vi "Car Wash.vi"() -> ()   [LabVIEW 2017]
uses:
  Bundyra/support/Message Queue/Message Queue.lvlib
  Bundyra/Boiler/Boiler.lvlib
  <vilib>/Utility/error.llb/Error Cluster From Error Code.vi
  <vilib>/ErrorRing/Error Ring.xnode
  Bundyra/Boiler/Boiler References.ctl
  Car Wash Data.ctl
  Bundyra/support/Message Queue/Message Cluster.ctl
  Bundyra/support/Message Queue/All Message Queues.ctl
  Bundyra/Boiler/Boiler Configuration.ctl
  Notifiers.ctl
panel:
  in  "Notifiers":T1
  in  "Boiler Configuration":T2
  in  "Message Queues":T3
  in  "error in":errorcluster
  out "error out":errorcluster
  in  "Simulate Failure":bool
  out "Vehicle Postion":bool
  out "Air Dry":bool
  out "Tire Shine Foam":bool
  out "Spot Free Rinse":bool
  out "Low Pressure  Wax":bool
  out "High Pressure Wash":bool
  out "Pre-soak":bool
  out "Bug Remover":bool
  out "Under Body Wash":bool
  # "Wash entry"
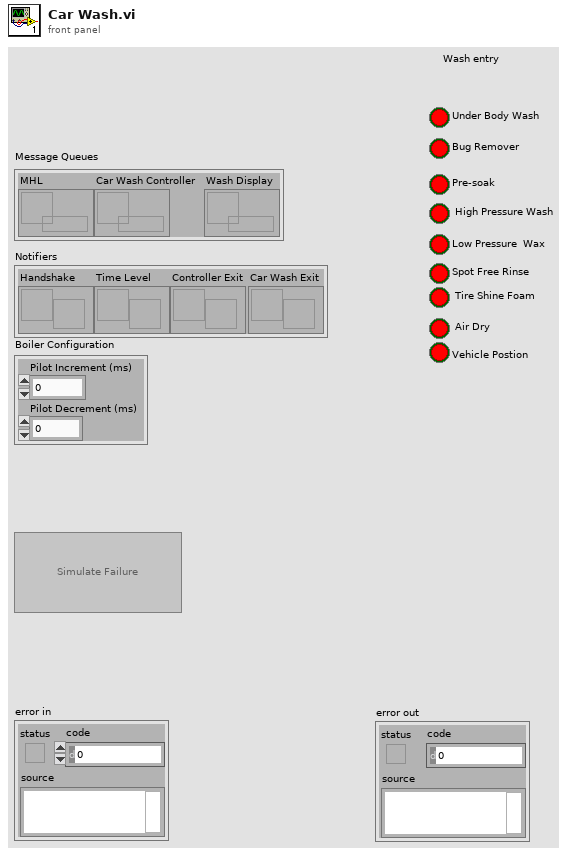
[diagram p1: front panel]
types:
  T1 = typedef "Notifiers.ctl" = cluster{"Handshake":refnum<notifier>, "Time Level":refnum<notifier>, "Controller Exit":refnum<notifier>, "Car Wash Exit":refnum<notifier>}
  T2 = typedef "Boiler.lvlib/Boiler Configuration.ctl" = cluster{"Pilot Increment (ms)":u32, "Pilot Decrement (ms)":u32}
  T3 = typedef "Message Queue.lvlib/All Message Queues.ctl" = cluster{"MHL":refnum<queue>, "Car Wash Controller":refnum<queue>, "Wash Display":refnum<queue>}
  T4 = typedef "Boiler.lvlib/Car Wash Data.ctl" = cluster{"Car Wash  References":T5, "Under Body Wash":bool, "Bug Remover":bool, "Pre-soak":bool, " High Pressure Wash":bool, "Low Pressure  Wax":bool, "Spot Free Rinse":bool, " Tire Shine Foam":bool, " Air Dry":bool, "Vehicle Position":bool}
  T5 = typedef "Boiler.lvlib/Boiler References.ctl" = cluster{"Simulate Failure":refnum<vi>}
  T6 = enum8{"Enabled", "Disabled", "Disabled and Grayed Out"}
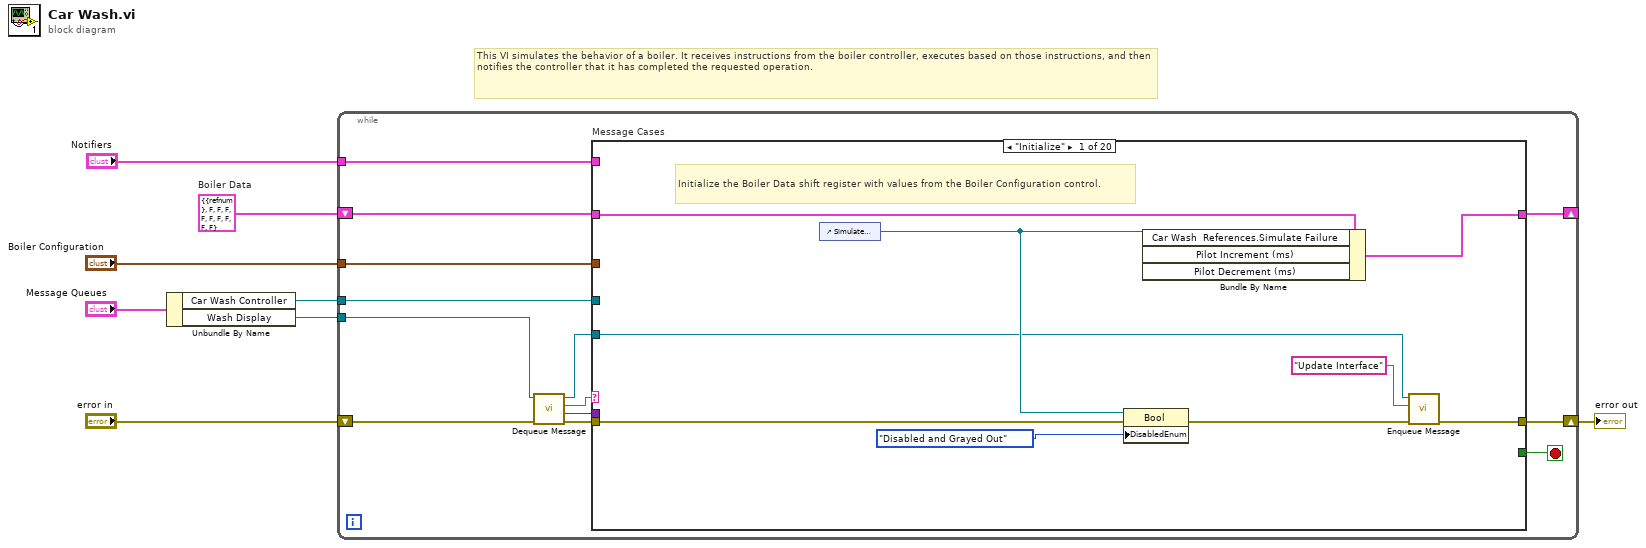
[diagram p0: block diagram]
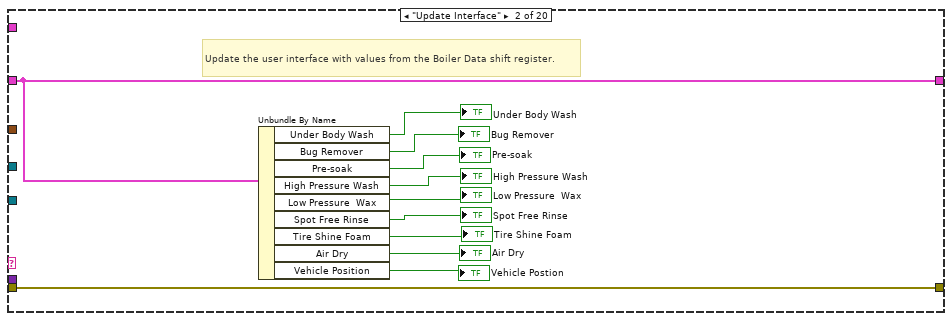
[diagram p2: hidden frame]
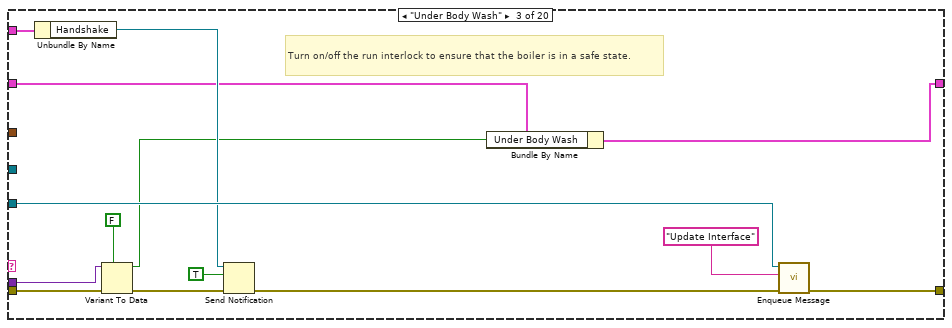
[diagram p3: hidden frame]
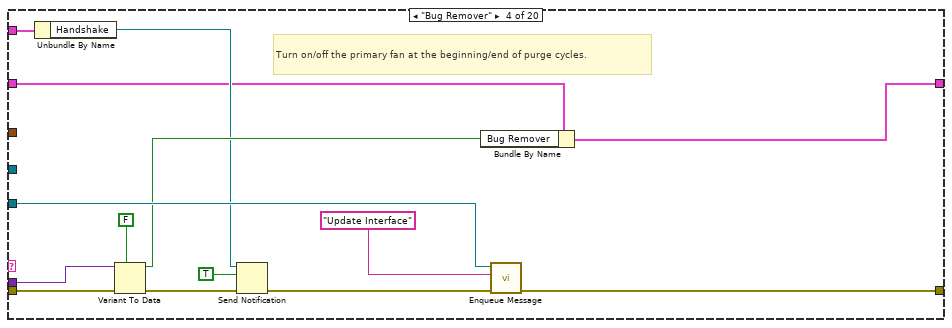
[diagram p4: hidden frame]
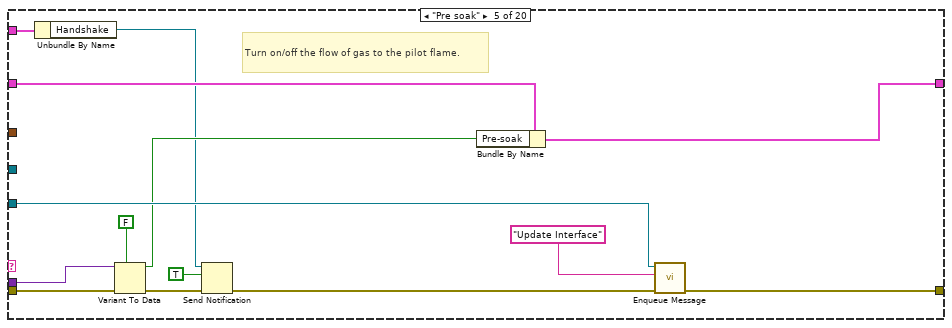
[diagram p5: hidden frame]
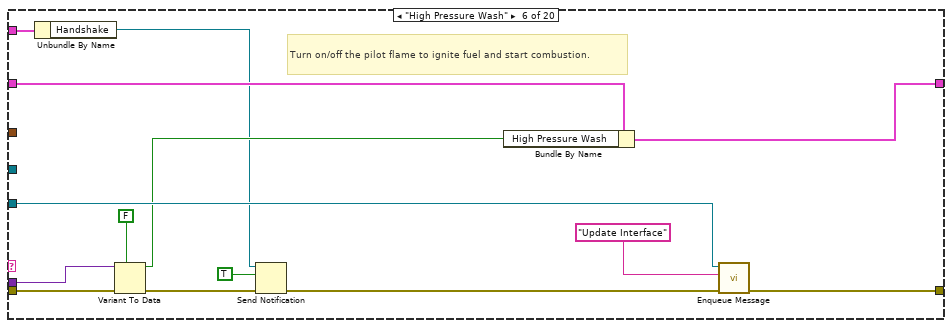
[diagram p6: hidden frame]
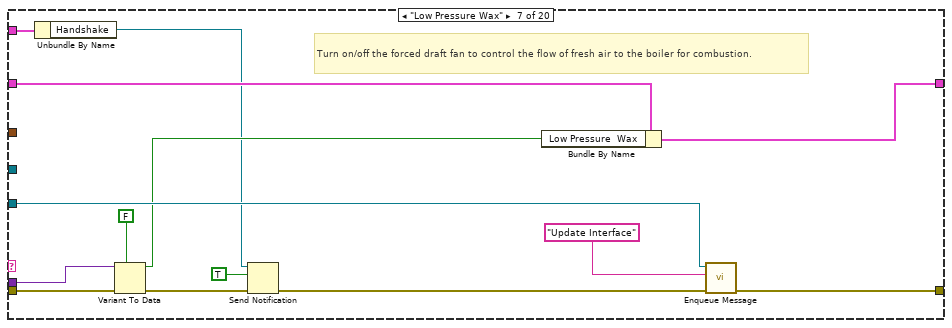
[diagram p7: hidden frame]
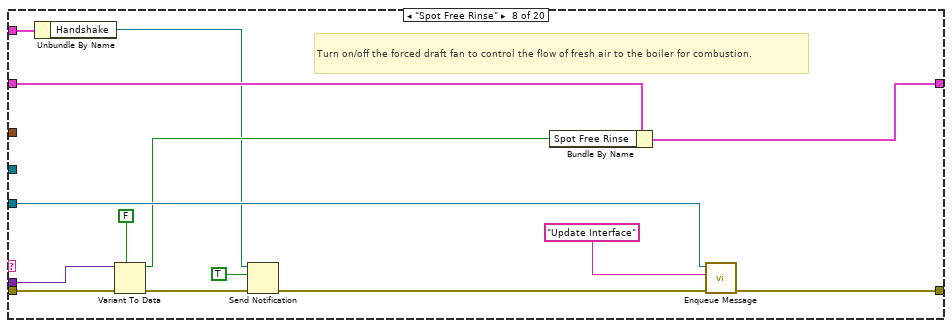
[diagram p8: hidden frame]
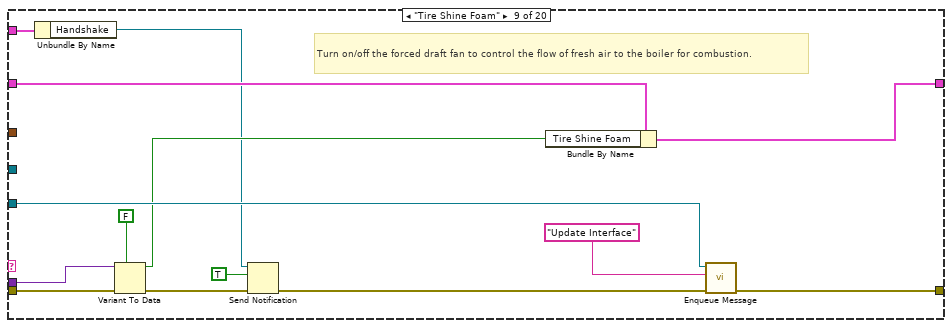
[diagram p9: hidden frame]
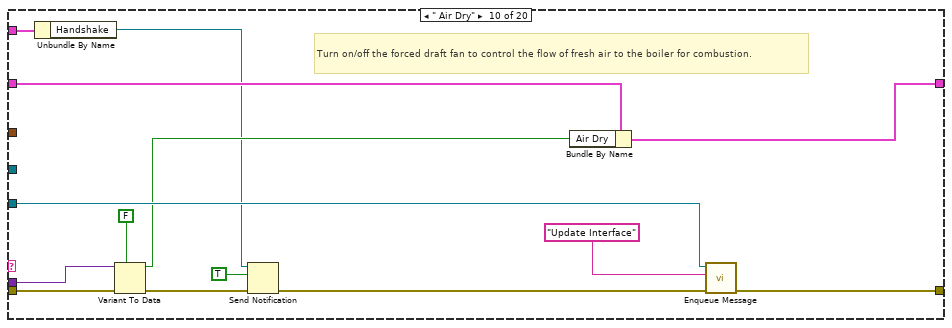
[diagram p10: hidden frame]
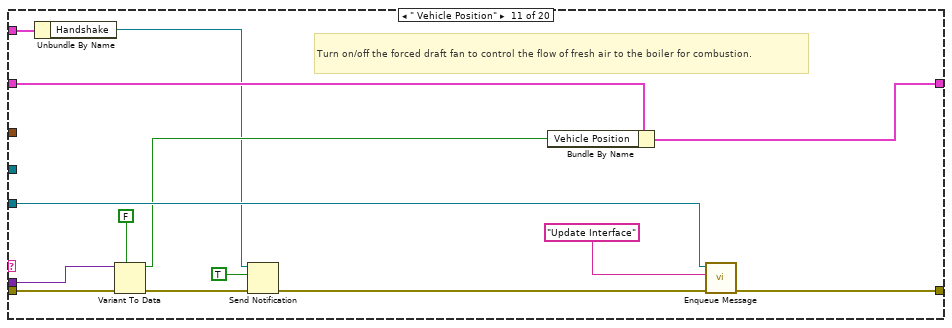
[diagram p11: hidden frame]
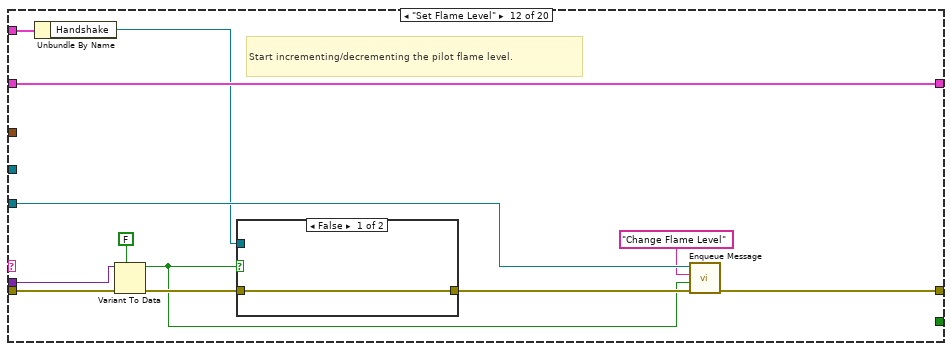
[diagram p12: hidden frame]
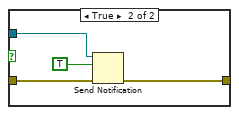
[diagram p13: hidden frame]
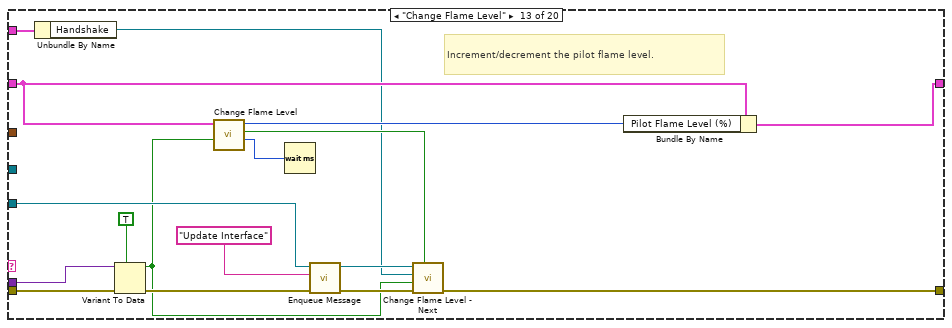
[diagram p14: hidden frame]
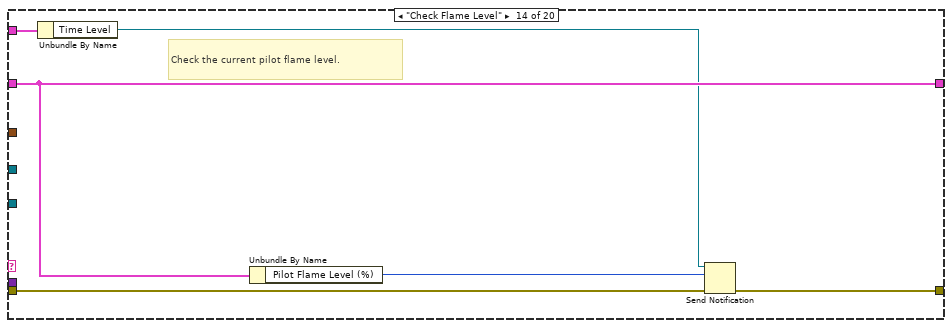
[diagram p15: hidden frame]
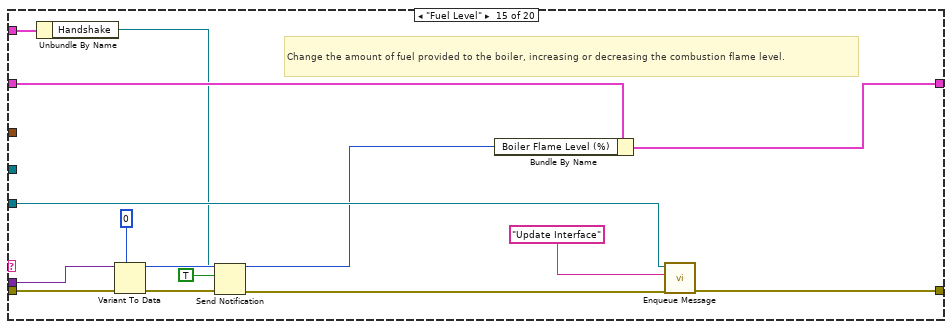
[diagram p16: hidden frame]
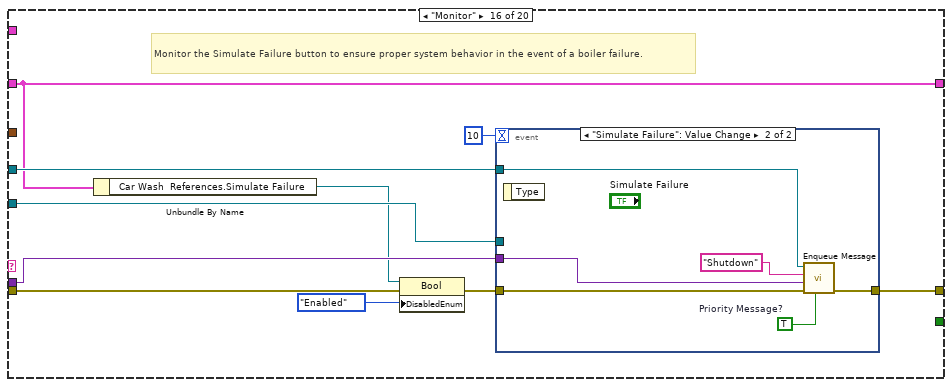
[diagram p17: hidden frame]
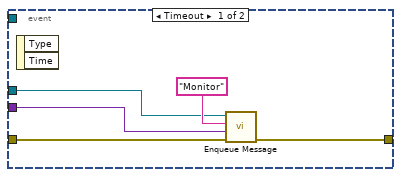
[diagram p18: hidden frame]
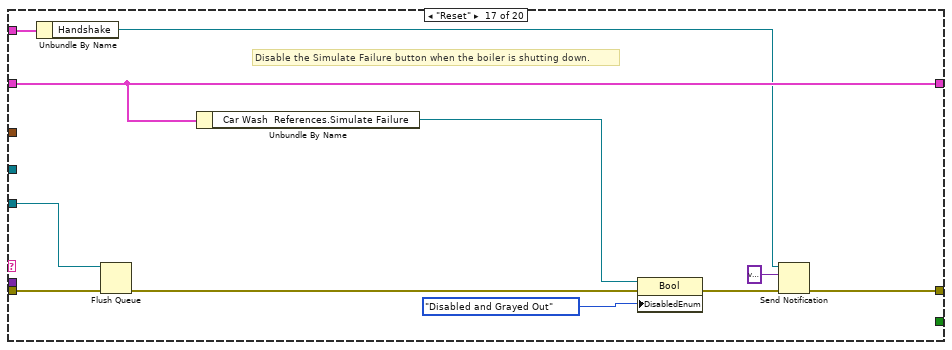
[diagram p19: hidden frame]
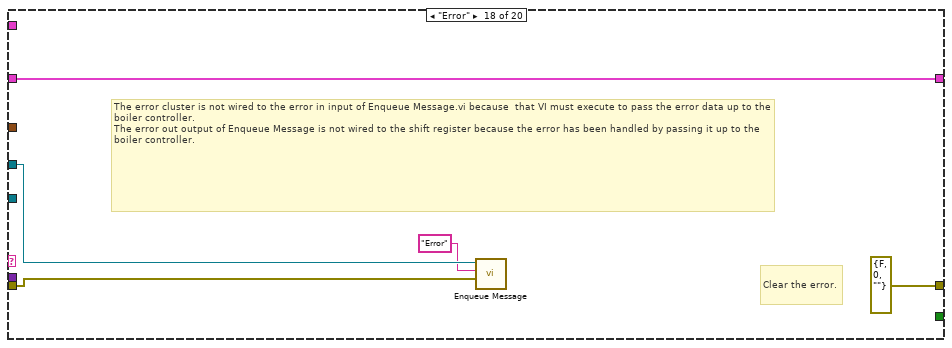
[diagram p20: hidden frame]
diagram:
  w7 = T4 {"Car Wash  References"={"Simulate Failure"=refnum}, "Under Body Wash"=FALSE, "Bug Remover"=FALSE, "Pre-soak"=FALSE, " High Pressure Wash"=FALSE, "Low Pressure  Wax"=FALSE, "Spot Free Rinse"=FALSE, " Tire Shine Foam"=FALSE, " Air Dry"=FALSE, "Vehicle Position"=FALSE}  # Boiler Data
  # "This VI simulates the behavior of a boiler. It receives instructions from the boiler controller, executes based on those instructions, and then notifies the controller that it has completed the requested operation."
  n1 = Unbundle By Name("Message Queues") -> ("Car Wash Controller"=w4:refnum<queue>, "Wash Display"=w3:refnum<queue>)
  n2 = while {
    tunnel: w3 -> [w12]
    shift-right: [w20] -> _
    shift-left: w7 -> [w21]
    shift-right: [w18] -> w8
    shift-left: "error in" -> [w17]
    tunnel: w4 -> [w11]
    tunnel: "Notifiers" -> [w10]
    tunnel: "Boiler Configuration" -> [w9]
    stop <- w19 stop-if-true
    n3 = call "Dequeue Message.vi"("error in (no error)"=w17, "Message Queue"=w12) -> ("error out"=w16:errorcluster, "Message Data"=w14:variant, "Message"=w15:string, "dup Message Queue"=w13:refnum<queue>)  [unwired: 6 in]
    n4 = case "Message Cases" shown="\"Initialize\"" w15 {
      selector: w15 -> [_ _ _ _ _ _ _ _ _ _ _ _ _ _ _ _ _ _ _ w269]
      tunnel: w13 -> [w24 _ w55 w65 w79 w93 w107 w121 w135 w149 w163 w177 w198 _ w218 w230 w250 _ w267 _]
      tunnel: w16 -> [w23 w41 w54 w67 w81 w95 w109 w123 w137 w151 w165 w174 w200 w204 w220 w222 w249 w255 w264 w275]
      tunnel: [w25 w41 w49 w61 w73 w87 w101 w115 w129 w143 w157 w178 w189 w207 w211 w223 w247 errorcluster {"status"=FALSE, "code"=0, "source"=""} ("error out") w263 w274] -> w18
      tunnel: w21 -> [w28 w40 w44 w57 w78 w92 w106 w120 w134 w148 w162 w179 w197 w206 w216 w224 w252 w258 w266 w276]
      tunnel: [w29 w40 w42 w56 w77 w91 w104 w118 w132 w146 w160 w179 w196 w206 w214 w224 w252 w258 w266 w276] -> w20
      tunnel: [_ _ _ _ _ _ _ _ _ _ _ _ _ _ _ _ _ _ TRUE _] -> w19
      tunnel: w14 -> [_ _ w52 w66 w80 w94 w108 w122 w136 w150 w164 w173 w199 _ w219 w228 _ _ _ _]
      tunnel: w11 -> [_ _ _ _ _ _ _ _ _ _ _ _ _ _ _ w229 _ w257 _ _]
      tunnel: w10 -> [_ _ w47 w60 w72 w86 w100 w114 w128 w142 w156 w169 w188 w205 w210 _ w246 _ w262 w272]
      tunnel: w9 -> [_ _ _ _ _ _ _ _ _ _ _ _ _ _ _ _ _ _ _ _]
      frame "Initialize" {
        # "Initialize the Boiler Data shift register with values from the Boiler Configuration control."
        n5 = control-ref of="Simulate Failure"() -> (w27:refnum<vi>)
        n6 = property class="Bool"(reference=w27, error in=w23, "DisabledEnum"=T6."Disabled and Grayed Out" ("Disabled")) -> (error out=w22:errorcluster)  [unwired: 1 out]
        n7 = Bundle By Name(cluster=w28, "Car Wash  References.Simulate Failure"=w27) -> (w29:T4)  [unwired: 2 in]
        n8 = call "Enqueue Message.vi"("error in (no error)"=w22, "Message"="Update Interface", "Message Queue"=w24) -> ("error out"=w25:errorcluster)  [unwired: 7 in, 1 out]
      }
      frame "Update Interface" {
        # "Update the user interface with values from the Boiler Data shift register."
        n9 = Unbundle By Name(w40) -> ("Under Body Wash"=→"Under Body Wash":bool, "Bug Remover"=→"Bug Remover":bool, "Pre-soak"=→"Pre-soak":bool, "High Pressure Wash"=→"High Pressure Wash":bool, "Low Pressure  Wax"=→"Low Pressure  Wax":bool, "Spot Free Rinse"=→"Spot Free Rinse":bool, "Tire Shine Foam"=→"Tire Shine Foam":bool, "Air Dry"=→"Air Dry":bool, "Vehicle Position"=→"Vehicle Postion":bool)
      }
      frame "Under Body Wash" {
        # "Turn on/off the run interlock to ensure that the boiler is in a safe state."
        n10 = Unbundle By Name(w47) -> ("Handshake"=w45:refnum<notifier>)
        n11 = Variant To Data(error in=w54, type=FALSE ("Run Interlock"), Variant=w52) -> (data=w43:bool, error out=w50:errorcluster)
        n12 = Send Notification(notification=TRUE, notifier=w45, error in (no error)=w50) -> (error out=w48:errorcluster)  [unwired: 1 out]
        n13 = Bundle By Name(cluster=w44, "Under Body Wash"=w43) -> (w42:T4)
        n14 = call "Enqueue Message.vi"("error in (no error)"=w48, "Message"="Update Interface", "Message Queue"=w55) -> ("error out"=w49:errorcluster)  [unwired: 7 in, 1 out]
      }
      frame "Bug Remover" {
        # "Turn on/off the primary fan at the beginning/end of purge cycles."
        n15 = Unbundle By Name(w60) -> ("Handshake"=w58:refnum<notifier>)
        n16 = Variant To Data(error in=w67, type=FALSE ("Run Interlock"), Variant=w66) -> (data=w64:bool, error out=w63:errorcluster)
        n17 = Send Notification(notification=TRUE ("Run Interlock"), notifier=w58, error in (no error)=w63) -> (error out=w62:errorcluster)  [unwired: 1 out]
        n18 = Bundle By Name(cluster=w57, "Bug Remover"=w64) -> (w56:T4)
        n19 = call "Enqueue Message.vi"("error in (no error)"=w62, "Message"="Update Interface", "Message Queue"=w65) -> ("error out"=w61:errorcluster)  [unwired: 7 in, 1 out]
      }
      frame "Pre soak" {
        # "Turn on/off the flow of gas to the pilot flame."
        n20 = Unbundle By Name(w72) -> ("Handshake"=w70:refnum<notifier>)
        n21 = Variant To Data(error in=w81, type=FALSE ("Run Interlock"), Variant=w80) -> (data=w76:bool, error out=w75:errorcluster)
        n22 = Send Notification(notification=TRUE ("Run Interlock"), notifier=w70, error in (no error)=w75) -> (error out=w74:errorcluster)  [unwired: 1 out]
        n23 = Bundle By Name(cluster=w78, "Pre-soak"=w76) -> (w77:T4)
        n24 = call "Enqueue Message.vi"("error in (no error)"=w74, "Message"="Update Interface", "Message Queue"=w79) -> ("error out"=w73:errorcluster)  [unwired: 7 in, 1 out]
      }
      frame "High Pressure Wash" {
        # "Turn on/off the pilot flame to ignite fuel and start combustion."
        n25 = Unbundle By Name(w86) -> ("Handshake"=w84:refnum<notifier>)
        n26 = Variant To Data(error in=w95, type=FALSE ("Run Interlock"), Variant=w94) -> (data=w90:bool, error out=w89:errorcluster)
        n27 = Send Notification(notification=TRUE ("Run Interlock"), notifier=w84, error in (no error)=w89) -> (error out=w88:errorcluster)  [unwired: 1 out]
        n28 = Bundle By Name(cluster=w92, "High Pressure Wash"=w90) -> (w91:T4)
        n29 = call "Enqueue Message.vi"("error in (no error)"=w88, "Message"="Update Interface", "Message Queue"=w93) -> ("error out"=w87:errorcluster)  [unwired: 7 in, 1 out]
      }
      frame "Low Pressure Wax" {
        # "Turn on/off the forced draft fan to control the flow of fresh air to the boiler for combustion."
        n30 = Unbundle By Name(w100) -> ("Handshake"=w98:refnum<notifier>)
        n31 = Variant To Data(error in=w109, type=FALSE ("Run Interlock"), Variant=w108) -> (data=w105:bool, error out=w103:errorcluster)
        n32 = Send Notification(notification=TRUE ("Run Interlock"), notifier=w98, error in (no error)=w103) -> (error out=w102:errorcluster)  [unwired: 1 out]
        n33 = Bundle By Name(cluster=w106, "Low Pressure  Wax"=w105) -> (w104:T4)
        n34 = call "Enqueue Message.vi"("error in (no error)"=w102, "Message"="Update Interface", "Message Queue"=w107) -> ("error out"=w101:errorcluster)  [unwired: 7 in, 1 out]
      }
      frame "Spot Free Rinse" {
        # "Turn on/off the forced draft fan to control the flow of fresh air to the boiler for combustion."
        n35 = Unbundle By Name(w114) -> ("Handshake"=w112:refnum<notifier>)
        n36 = Variant To Data(error in=w123, type=FALSE ("Run Interlock"), Variant=w122) -> (data=w119:bool, error out=w117:errorcluster)
        n37 = Send Notification(notification=TRUE ("Run Interlock"), notifier=w112, error in (no error)=w117) -> (error out=w116:errorcluster)  [unwired: 1 out]
        n38 = Bundle By Name(cluster=w120, "Spot Free Rinse"=w119) -> (w118:T4)
        n39 = call "Enqueue Message.vi"("error in (no error)"=w116, "Message"="Update Interface", "Message Queue"=w121) -> ("error out"=w115:errorcluster)  [unwired: 7 in, 1 out]
      }
      frame "Tire Shine Foam" {
        # "Turn on/off the forced draft fan to control the flow of fresh air to the boiler for combustion."
        n40 = Unbundle By Name(w128) -> ("Handshake"=w126:refnum<notifier>)
        n41 = Variant To Data(error in=w137, type=FALSE ("Run Interlock"), Variant=w136) -> (data=w133:bool, error out=w131:errorcluster)
        n42 = Send Notification(notification=TRUE ("Run Interlock"), notifier=w126, error in (no error)=w131) -> (error out=w130:errorcluster)  [unwired: 1 out]
        n43 = Bundle By Name(cluster=w134, "Tire Shine Foam"=w133) -> (w132:T4)
        n44 = call "Enqueue Message.vi"("error in (no error)"=w130, "Message"="Update Interface", "Message Queue"=w135) -> ("error out"=w129:errorcluster)  [unwired: 7 in, 1 out]
      }
      frame " Air Dry" {
        # "Turn on/off the forced draft fan to control the flow of fresh air to the boiler for combustion."
        n45 = Unbundle By Name(w142) -> ("Handshake"=w140:refnum<notifier>)
        n46 = Variant To Data(error in=w151, type=FALSE ("Run Interlock"), Variant=w150) -> (data=w147:bool, error out=w145:errorcluster)
        n47 = Send Notification(notification=TRUE ("Run Interlock"), notifier=w140, error in (no error)=w145) -> (error out=w144:errorcluster)  [unwired: 1 out]
        n48 = Bundle By Name(cluster=w148, "Air Dry"=w147) -> (w146:T4)
        n49 = call "Enqueue Message.vi"("error in (no error)"=w144, "Message"="Update Interface", "Message Queue"=w149) -> ("error out"=w143:errorcluster)  [unwired: 7 in, 1 out]
      }
      frame " Vehicle Position" {
        # "Turn on/off the forced draft fan to control the flow of fresh air to the boiler for combustion."
        n50 = Unbundle By Name(w156) -> ("Handshake"=w154:refnum<notifier>)
        n51 = Variant To Data(error in=w165, type=FALSE ("Run Interlock"), Variant=w164) -> (data=w161:bool, error out=w159:errorcluster)
        n52 = Send Notification(notification=TRUE ("Run Interlock"), notifier=w154, error in (no error)=w159) -> (error out=w158:errorcluster)  [unwired: 1 out]
        n53 = Bundle By Name(cluster=w162, "Vehicle Position"=w161) -> (w160:T4)
        n54 = call "Enqueue Message.vi"("error in (no error)"=w158, "Message"="Update Interface", "Message Queue"=w163) -> ("error out"=w157:errorcluster)  [unwired: 7 in, 1 out]
      }
      frame "Set Flame Level" {
        # "Start incrementing/decrementing the pilot flame level."
        n55 = Unbundle By Name(w169) -> ("Handshake"=w168:refnum<notifier>)
        n56 = Variant To Data(error in=w174, type=FALSE ("Run Interlock"), Variant=w173) -> (data=w170:bool, error out=w172:errorcluster)
        n57 = case shown="False" w170 {
          tunnel: w172 -> [w180 w184]
          tunnel: [w180 w183] -> w171
          tunnel: w168 -> [_ w181]
          frame False {
          }
          frame True {
            n58 = Send Notification(notification=TRUE ("Run Interlock"), notifier=w181, error in (no error)=w184) -> (error out=w183:errorcluster)  [unwired: 1 out]
          }
        }
        n59 = call "Enqueue Message.vi"("error in (no error)"=w171, "Message Data"=w170, "Message"="Change Flame Level", "Message Queue"=w177) -> ("error out"=w178:errorcluster)  [unwired: 6 in, 1 out]
      }
      frame "Change Flame Level" {
        # "Increment/decrement the pilot flame level."
        n60 = Unbundle By Name(w188) -> ("Handshake"=w186:refnum<notifier>)
        n61 = Variant To Data(error in=w200, type=TRUE, Variant=w199) -> (data=w185:bool, error out=w192:errorcluster)
        n62 = call "Change Flame Level.vi"("Increment?"=w185, "Boiler Data"=w197) -> ("Time Increment"=w193:u32, "Limit?"=w187:bool, "Flame Level"=w194:u32)  [unwired: 7 in]
        n63 = Wait (ms)(milliseconds to wait=w193) -> ()  [unwired: 1 out]
        n64 = call "Enqueue Message.vi"("error in (no error)"=w192, "Message"="Update Interface", "Message Queue"=w198) -> ("error out"=w190:errorcluster, "dup Message Queue"=w191:refnum<queue>)  [unwired: 7 in]
        n65 = call "Change Flame Level - Next.vi"("Limit?"=w187, "error in"=w190, "Increment?"=w185, "Handshake"=w186, "Boiler Queue in"=w191) -> ("error out"=w189:errorcluster)  [unwired: 6 in]
        n66 = Bundle By Name(cluster=w197, "Pilot Flame Level (%)"=w194) -> (w196:T4)
      }
      frame "Check Flame Level" {
        # "Check the current pilot flame level."
        n67 = Unbundle By Name(w205) -> ("Time Level"=w202:refnum<notifier>)
        n68 = Unbundle By Name(w206) -> ("Pilot Flame Level (%)"=w203:u32)
        n69 = Send Notification(notification=w203, notifier=w202, error in (no error)=w204) -> (error out=w207:errorcluster)  [unwired: 1 out]
      }
      frame "Fuel Level" {
        # "Change the amount of fuel provided to the boiler, increasing or decreasing the combustion flame level."
        n70 = Unbundle By Name(w210) -> ("Handshake"=w208:refnum<notifier>)
        n71 = Variant To Data(error in=w220, type=u32 0, Variant=w219) -> (data=w215:u32, error out=w213:errorcluster)
        n72 = Send Notification(notification=TRUE ("Run Interlock"), notifier=w208, error in (no error)=w213) -> (error out=w212:errorcluster)  [unwired: 1 out]
        n73 = Bundle By Name(cluster=w216, "Boiler Flame Level (%)"=w215) -> (w214:T4)
        n74 = call "Enqueue Message.vi"("error in (no error)"=w212, "Message"="Update Interface", "Message Queue"=w218) -> ("error out"=w211:errorcluster)  [unwired: 7 in, 1 out]
      }
      frame "Monitor" {
        # "Monitor the Simulate Failure button to ensure proper system behavior in the event of a boiler failure."
        n75 = Unbundle By Name(w224) -> ("Car Wash  References.Simulate Failure"=w227:refnum<vi>)
        n76 = property class="Bool"(reference=w227, error in=w222, "DisabledEnum"=T6."Enabled" ("Disabled")) -> (error out=w225:errorcluster)  [unwired: 1 out]
        n77 = event shown="[1] \"Simulate Failure\": Value Change" {
          selector: _ -> [_ _]
          dyn-events: _ -> [_ _]
          timeout: 10 -> [_ _]
          tunnel: w225 -> [w235 w239]
          tunnel: [w234 w240] -> w223
          tunnel: w230 -> [w233 _]
          tunnel: w229 -> [_ w242]
          tunnel: w228 -> [w232 w238]
          event Timeout {
            n78 = event-data() -> ()  [unwired: 1 in, 2 out]
            n79 = call "Enqueue Message.vi"("error in (no error)"=w235, "Message Data"=w232, "Message"="Monitor", "Message Queue"=w233) -> ("error out"=w234:errorcluster)  [unwired: 6 in, 1 out]
          }
          event "Simulate Failure": Value Change {
            w237 = TRUE  # Priority Message?
            n80 = event-data() -> ()  [unwired: 1 in, 1 out]
            n81 = call "Enqueue Message.vi"("Priority Message? (F)"=w237, "error in (no error)"=w239, "Message Data"=w238, "Message"="Shutdown", "Message Queue"=w242) -> ("error out"=w240:errorcluster)  [unwired: 5 in, 1 out]
          }
        }
      }
      frame "Reset" {
        # "Disable the Simulate Failure button when the boiler is shutting down."
        n82 = Unbundle By Name(w246) -> ("Handshake"=w245:refnum<notifier>)
        n83 = Flush Queue(queue=w250, error in (no error)=w249) -> (error out=w243:errorcluster)  [unwired: 2 out]
        n84 = Unbundle By Name(w252) -> ("Car Wash  References.Simulate Failure"=w251:refnum<vi>)
        n85 = property class="Bool"(reference=w251, error in=w243, "DisabledEnum"=T6."Disabled and Grayed Out" ("Disabled")) -> (error out=w248:errorcluster)  [unwired: 1 out]
        n86 = Send Notification(notification=variant, notifier=w245, error in (no error)=w248) -> (error out=w247:errorcluster)  [unwired: 1 out]
      }
      frame "Error" {
        # "Clear the error."
        # "The error cluster is not wired to the error in input of Enqueue Message.vi because  that VI must execute to pass the error data up to the boiler controller.\nThe error out output of Enqueue Message is not wired to the shift register because the error has been handled by passing it up to the boiler controller."
        n87 = call "Enqueue Message.vi"("Message Data"=w255, "Message"="Error", "Message Queue"=w257) -> ()  [unwired: 7 in, 2 out]
      }
      frame "Exit" {
        # "Shut down the boiler. Release the queue."
        # "Stop the VI"
        n88 = Unbundle By Name(w262) -> ("Car Wash Exit"=w260:refnum<notifier>)
        n89 = Release Queue(queue=w267, error in (no error)=w264) -> (error out=w261:errorcluster)  [unwired: 1 in, 2 out]
        n90 = Send Notification(notification=variant, notifier=w260, error in (no error)=w261) -> (error out=w263:errorcluster)  [unwired: 1 out]
      }
      frame Default {
        # "'Default' case only runs if there is a message that isn't defined in any of the other cases.  Output a programming error."
        n91 = Unbundle By Name(w272) -> ("Handshake"=w271:refnum<notifier>)
        n92 = Send Notification(notification=variant, notifier=w271, error in (no error)=w275) -> (error out=w273:errorcluster)  [unwired: 1 out]
        n93 = xnode "Error Ring"("parameter 0"=w269) -> ("error out"=w268:errorcluster)
        n94 = Merge Errors(w268, w273) -> (w274:errorcluster)
      }
    }
  }
  "error out" <- w8
